vi "publish -- glue -- number V2.vi"(7 "publisher action":T1, 8 "request event IN":refnum<user-event>) -> (0 "request event":refnum<user-event>, 2 "Event Registration Refnum out":refnum<event-registration>)   [LabVIEW 2018]
uses:
  publisher action.ctl
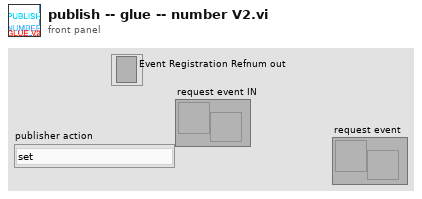
[diagram p1: front panel]
types:
  T1 = typedef "publisher action.ctl" = enum16{"set", "get", "init", "check"}
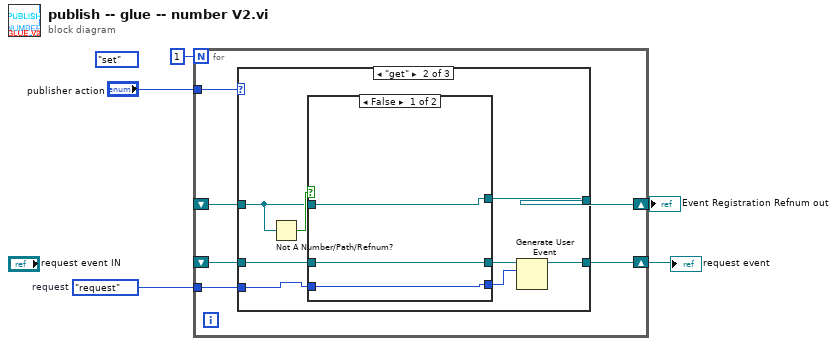
[diagram p0: block diagram]
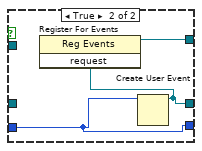
[diagram p3: hidden frame]
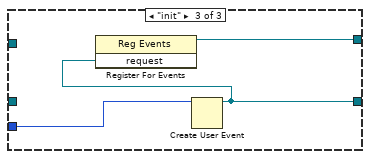
[diagram p4: hidden frame]
diagram:
  w2 = enum16{"request"}."request"  # request
  (unwired) publisher_action."set" ("publisher action")
  n1 = for {
    N: 1 -> [_]
    shift-right: [w11] -> w5
    shift-left: _ -> [w9]
    tunnel: "publisher action" -> [w10]
    tunnel: w2 -> [w8]
    shift-right: [w7] -> w1
    shift-left: _ -> [w6]
    n2 = case shown="\"get\"" w10 {
      tunnel: [w13 w21 w29] -> w11
      tunnel: w9 -> [w13 w14 _]
      tunnel: w8 -> [_ w20 w30]
      tunnel: [w12 w16 w28] -> w7
      tunnel: w6 -> [w12 w15 _]
      frame "check", Default {
      }
      frame "get" {
        n3 = Not A Number/Path/Refnum?(number/path/refnum=w15) -> (NaN/Path/Refnum?=w17:bool)
        n4 = case shown="False" w17 {
          tunnel: w20 -> [w22 w27]
          tunnel: [w23 w26] -> w19
          tunnel: [w22 w27] -> w18
          tunnel: [w24 w25] -> w16
          tunnel: w15 -> [w24 _]
          tunnel: w14 -> [w23 _]
          frame False {
          }
          frame True {
            n5 = Create User Event(user event datatype=w27) -> (user event=w26:refnum<user-event>)  [unwired: 1 in, 1 out]
            n6 = register-events(w26) -> (reference out=w25:refnum<event-registration>)  [unwired: 2 in, 1 out]
          }
        }
        n7 = Generate User Event(user event=w19, event data cluster=w18) -> (user event out=w21:refnum<user-event>)  [unwired: 2 in, 1 out]
      }
      frame "init" {
        n8 = Create User Event(user event datatype=w30) -> (user event=w29:refnum<user-event>)  [unwired: 1 in, 1 out]
        n9 = register-events(w29) -> (reference out=w28:refnum<event-registration>)  [unwired: 2 in, 1 out]
      }
    }
  }
  "request event" <- w5
  "Event Registration Refnum out" <- w1
